vi "LinearSystemLoop_FlyWheel_Pack_Ctrl.vi"(8 "Max Ctrl Out V":dbl=12.0, 9 "Vel Ctrl Tol Rad/Sec":dbl=0.1, 10 "Vel Meas Std Dev Rad/Sec":dbl=0.1, 11 "Vel Model Std Dev Rad/Sec":dbl=0.5) -> (3 "LinearSystemLoop_FlyWheel_Ctrl_Params":T1)   [LabVIEW 2019, in "Trajectory_Library.lvlib"]
doc: "Pack the control parameters for a flywheel linear system. \n\nThe flywheel linear system definition is:\n - States\n - angular velocity (Rad/Sec)\n - Inputs:\n - motor voltage\n - Outputs:\n - angular velocity (rad/sec)\n\nInputs:\n - Vel Model Std Dev -- double -- Standard deviation for modeled velocity (rad/sec)\n - Vel Meas Std Dev -- double -- Standard deviation for measured velocity (rad/sec)\n - Vel Ctrl Tol Std Dev -- double -- Control tolerance for velocity (rad/sec)\n - Max Ctrl Out -- double -- Maximum control output (Default: 12) (volts)\n\nOutputs:\n - LinearSystemLoop Flywheel Ctrl Params -- cluster -- Packed control parameters"
uses:
  Trajectory_Library.lvlib
  TypeDef/LINEAR_SYSTEM_LOOP_FLYWHEEL_CTRL_PARAMS.CTL
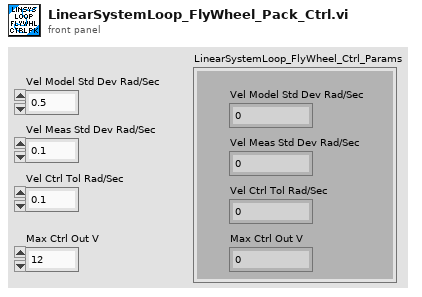
[diagram p1: front panel]
types:
  T1 = typedef "Trajectory_Library.lvlib/LINEAR_SYSTEM_LOOP_FLYWHEEL_CTRL_PARAMS.CTL" = cluster{"Vel Model Std Dev Rad/Sec":dbl, "Vel Meas Std Dev Rad/Sec":dbl, "Vel Ctrl Tol Rad/Sec":dbl, "Max Ctrl Out V":dbl}
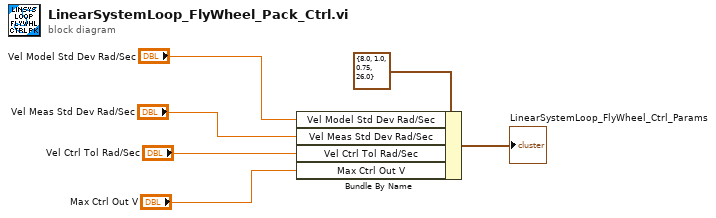
[diagram p0: block diagram]
diagram:
  n1 = Bundle By Name(cluster=T1 {"Vel Model Std Dev Rad/Sec"=8.0, "Vel Meas Std Dev Rad/Sec"=1.0, "Vel Ctrl Tol Rad/Sec"=0.75, "Max Ctrl Out V"=26.0} ("DCMotorSim_Model _Params"), "Vel Model Std Dev Rad/Sec"="Vel Model Std Dev Rad/Sec", "Vel Meas Std Dev Rad/Sec"="Vel Meas Std Dev Rad/Sec", "Vel Ctrl Tol Rad/Sec"="Vel Ctrl Tol Rad/Sec", "Max Ctrl Out V"="Max Ctrl Out V") -> (→"LinearSystemLoop_FlyWheel_Ctrl_Params":T1)
